vi "TCP Write.vi"(8 "error in (no error)":errorcluster, 9 "timeout":i32, 10 "data":u8[](array[numeric]), 11 "connection ID":refnum<k5>) -> (0 "error out":errorcluster, 1 "timed out?":bool)   [LabVIEW 2018, in "SubVIs.lvlib" / "TCP Shared Components.lvlib"]
doc: "This VI writes a set of data to a TCP connection and checks for errors. It is a wrapper for standard functionality."
uses:
  TCP Shared Components.lvlib
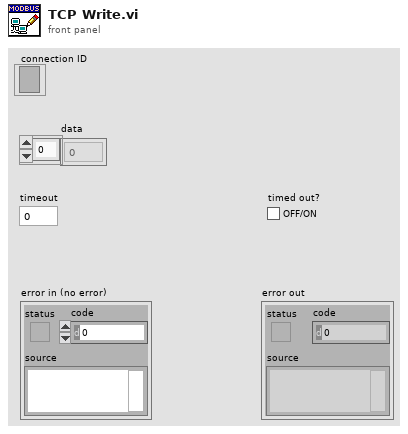
[diagram p1: front panel]
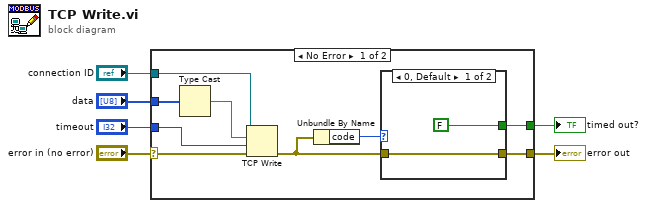
[diagram p0: block diagram]
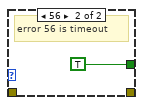
[diagram p2: hidden frame]
diagram:
  n1 = case shown="No Error" "error in (no error)" {
    selector: "error in (no error)" -> [w9 w19]
    tunnel: [w15 w19] -> w6
    tunnel: "timeout" -> [w14 _]
    tunnel: "data" -> [w13 _]
    tunnel: "connection ID" -> [w12 _]
    tunnel: [w7 _] -> w1
    frame No Error {
      n2 = Type Cast(x=w13) -> (*(type *) &x=w11:string)  [unwired: 1 in]
      n3 = TCP Write(connection ID=w12, data in=w11, error in (no error)=w9, 9:w14) -> (error out=w10:errorcluster)  [unwired: 2 out]
      n4 = Unbundle By Name(w10) -> ("code"=w8:i32)
      n5 = case shown="0, Default" w8 {
        tunnel: w10 -> [w17 _]
        tunnel: [w17 _] -> w15
        tunnel: [FALSE TRUE] -> w7
        frame 0, Default {
        }
        frame 56 {
          # "error 56 is timeout"
        }
      }
    }
    frame Error {
    }
  }
  "error out" <- w6
  "timed out?" <- w1
